vi "test tdms write read simultaneously.vi"() -> ()   [LabVIEW 2020]
panel:
  out "Waveform Graph 2":cluster{"f0":dbl, "df":dbl, "magnitude":dbl[]}[](graph)
  out "Waveform Graph":dbl[][](graph)
  out "Array":dbl[][](array[numeric])
  in  "stop":bool
  out "Refnum out":refnum<k34>
  in  "save path":path
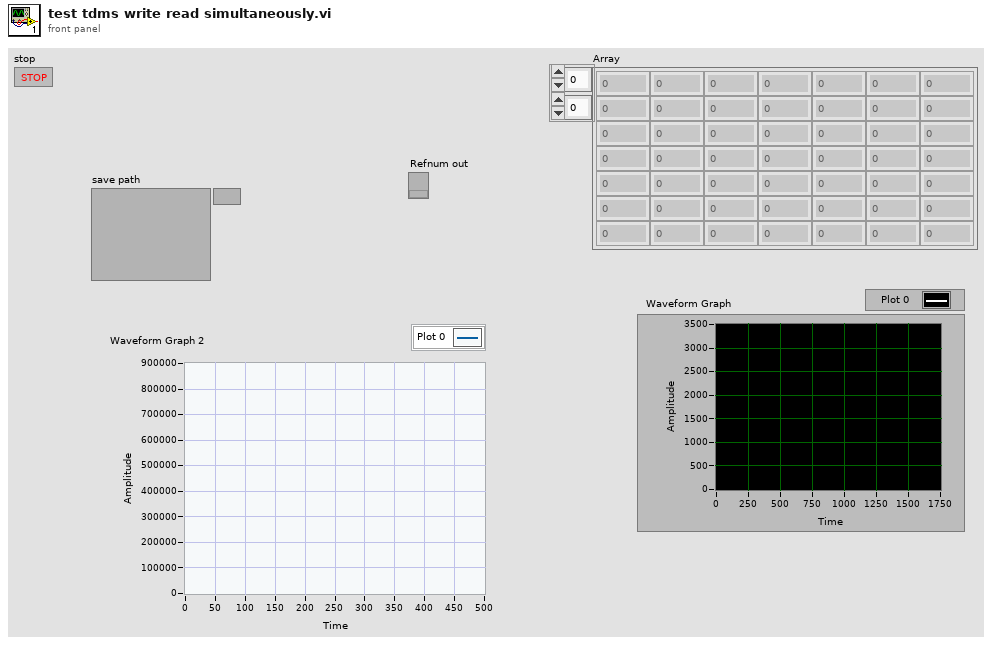
[diagram p1: front panel]
types:
  T1 = enum16{"open", "open or create", "create or replace", "create", "open (read-only)"}
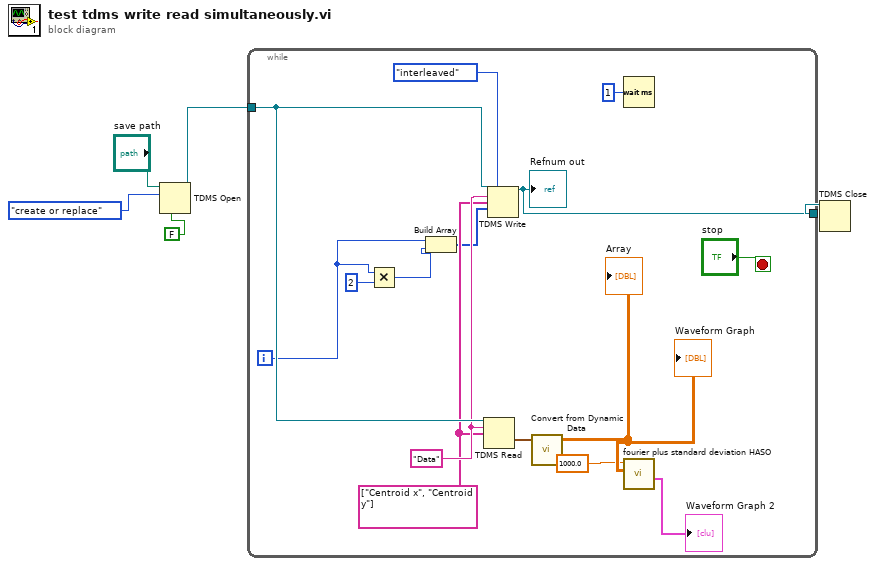
[diagram p0: block diagram]
diagram:
  n1 = TDMS Open(6:FALSE ("disable buffering (T)"), 10:T1."create or replace" ("operation"), 11:"save path") -> (3:w2:refnum<k34>)  [unwired: 4 in, 1 out]
  n2 = while {
    tunnel: w2 -> [w17]
    tunnel: [w14] -> w1
    i -> [w11]
    stop <- "stop" stop-if-true
    w15 = string[] ["Centroid x", "Centroid y"] ("channel name(s) in (Untitled)")
    w16 = "Data" ("group name in (Untitled)")
    n3 = Multiply(x=w11, y=2) -> (x*y=w10:i32)
    n4 = Build Array(w11, w10) -> (w13:i32[])
    n5 = TDMS Read(0:w17, 5:w16, 7:w15) -> (10:w12:waveform(dbl)[])  [unwired: 5 in, 5 out]
    n6 = TDMS Write(0:w17, 1:enum16{"decimated", "interleaved"}."interleaved" ("data layout (0:decimated)"), 5:w16, 7:w15, 9:w13) -> (4:w14:refnum<k34>)  [unwired: 1 in, 3 out]
    "Refnum out" <- w14
    n7 = call "Convert from Dynamic Data"("Dynamic Data Type"=w12) -> ("Array"=w8:dbl[][])  [unwired: 3 in]
    "Array" <- w8
    "Waveform Graph" <- w8
    n8 = Wait (ms)(milliseconds to wait=u32 1) -> ()  [unwired: 1 out]
    n9 = call "fourier plus standard deviation HASO.vi"("Array in"=w8, "rep rate (Hz)"=sgl 1000.0) -> ("Power spectral density"=→"Waveform Graph 2":cluster{"f0":dbl, "df":dbl, "magnitude":dbl[]}[])  [unwired: 7 in, 2 out]
  }
  n10 = TDMS Close(11:w1) -> ()  [unwired: 1 in, 2 out]
